vi "N Asymmetric Gaussians Fit Guess Parameters.vi"(8 "N":i32, 9 "Cursor X Array":dbl[](array[numeric]), 10 "Y Array":dbl[](array[numeric]), 11 "X Array":dbl[](array[numeric])) -> (1 "Guess Parameters Array":dbl[](array[numeric]), 2 "Y Array dup":dbl[](array[numeric]), 3 "X Array dup":dbl[](array[numeric]))   [LabVIEW 2019]
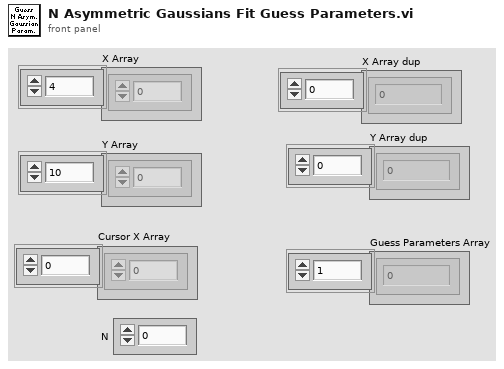
[diagram p1: front panel]
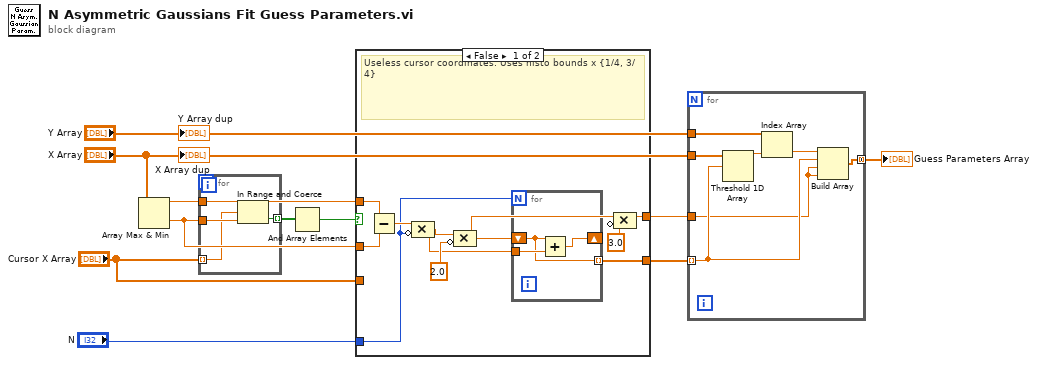
[diagram p0: block diagram]
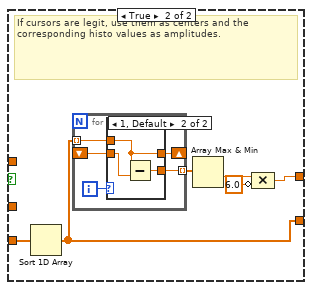
[diagram p2: hidden frame]
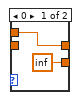
[diagram p3: hidden frame]
diagram:
  n1 = Array Max & Min(array="X Array") -> (max value=w4:dbl, min value=w3:dbl)  [unwired: 2 out]
  n2 = for {
    tunnel: w4 -> [w15]
    tunnel: w3 -> [w14]
    tunnel: "Cursor X Array" -> [w13] mode=indexing
    tunnel: [w12] -> w9 mode=indexing
    n3 = In Range and Coerce(upper limit=w15, x=w13, lower limit=w14) -> (In Range?=w12:bool)  [unwired: 1 out]
  }
  n4 = And Array Elements(Boolean array=w9) -> (logical AND=w1:bool)
  n5 = case shown="False" w1 {
    tunnel: "Cursor X Array" -> [_ w34]
    tunnel: [w19 w33] -> w7
    tunnel: [w17 w30] -> w5
    tunnel: w4 -> [w25 _]
    tunnel: w3 -> [w24 _]
    tunnel: "N" -> [w21 _]
    frame False {
      # "Useless cursor coordinates. Uses histo bounds x {1/4, 3/4}"
      n6 = Subtract(x=w25, y=w24) -> (x-y=w23:dbl)
      n7 = Compound Arithmetic op=MULTIPLY(w23, invert w21) -> (w20:dbl)
      n8 = Compound Arithmetic op=MULTIPLY(w20, invert 2.0 ("value")) -> (w18:dbl)
      n9 = for {
        N: w21 -> [_]
        shift-right: [w28] -> _
        shift-left: w18 -> [w26]
        tunnel: w20 -> [w27]
        tunnel: [w26] -> w19 mode=indexing
        n10 = Add(x=w26, y=w27) -> (x+y=w28:dbl)
      }
      n11 = Compound Arithmetic op=MULTIPLY(w18, invert 3.0 ("value")) -> (w17:dbl)
    }
    frame True {
      # "If cursors are legit, use them as centers and the corresponding histo values as amplitudes."
      n12 = Sort 1D Array(array=w34) -> (sorted array=w33:dbl[])
      n13 = for {
        tunnel: w33 -> [w37] mode=indexing
        shift-right: [w38] -> _
        shift-left: _ -> [w36]
        tunnel: [w35] -> w32 mode=indexing
        i -> [w39]
        n14 = case shown="1, Default" w39 {
          tunnel: [w41 w43] -> w38
          tunnel: w37 -> [w41 w43]
          tunnel: w36 -> [_ w44]
          tunnel: [inf w42] -> w35
          frame 0 {
          }
          frame 1, Default {
            n15 = Subtract(x=w43, y=w44) -> (x-y=w42:dbl)
          }
        }
      }
      n16 = Array Max & Min(array=w32) -> (min value=w31:dbl)  [unwired: 3 out]
      n17 = Compound Arithmetic op=MULTIPLY(w31, invert 6.0 ("value")) -> (w30:dbl)
    }
  }
  n18 = for {
    tunnel: "X Array" -> [w50]
    tunnel: "Y Array" -> [w49]
    tunnel: w7 -> [w47] mode=indexing
    tunnel: [w46] -> w6 mode=concatenating
    tunnel: w5 -> [w45]
    n19 = Threshold 1D Array(2:w47, 3:w50) -> (0:w51:dbl)  [unwired: 1 in]
    n20 = Index Array(array=w49, index=w51) -> (element=w48:dbl)
    n21 = Build Array(w48, w47, w45, w45) -> (w46:dbl[])
  }
  "Guess Parameters Array" <- w6
  "X Array dup" <- "X Array"
  "Y Array dup" <- "Y Array"
